vi "SLL DE Generate Plot LV2Global.vi"(7 "Option":T1=enum."Get Plot", 8 "error in (no error)":errorcluster, 9 "X-Scale":refnum<vi>, 10 "Plots":u16[](array[numeric]), 11 "Data Cluster":T3) -> (0 "error IO":errorcluster, 3 "Plot data array":T2(array[cluster]))   [LabVIEW 2009]
uses:
  Controls/SLL DE Get Plot LV2Global Parameters.ctl
  Controls/SLL DE Get Plot LV2Global Options.ctl
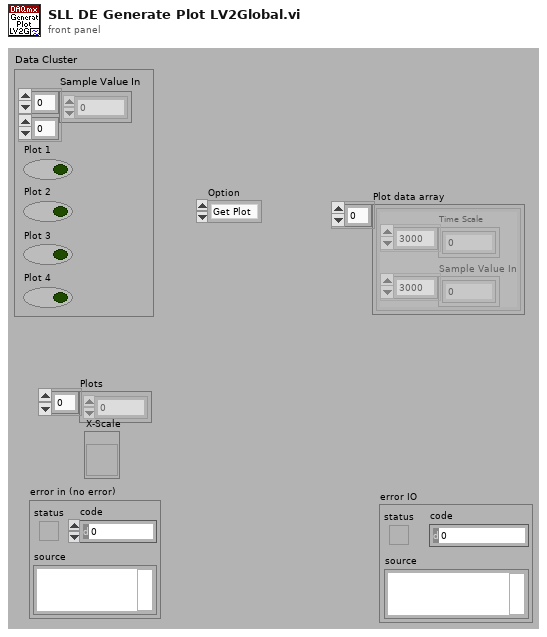
[diagram p1: front panel]
types:
  T1 = typedef "SLL DE Get Plot LV2Global Options.ctl" = enum16{"Init", "Get Plot", "Read Plot"}
  T2 = cluster{"Time Scale":sgl[], "Sample Value In":sgl[]}[]
  T3 = typedef "SLL DE Get Plot LV2Global Parameters.ctl" = cluster{"Sample Value In":sgl[][], "Plot 1":bool, "Plot 2":bool, "Plot 3":bool, "Plot 4":bool}
  T4 = cluster{"Sample Value In":sgl[], "Sample Value In":sgl[]}[]
  T5 = cluster{"Sample Value In":dbl[], "Sample Value In":sgl[]}
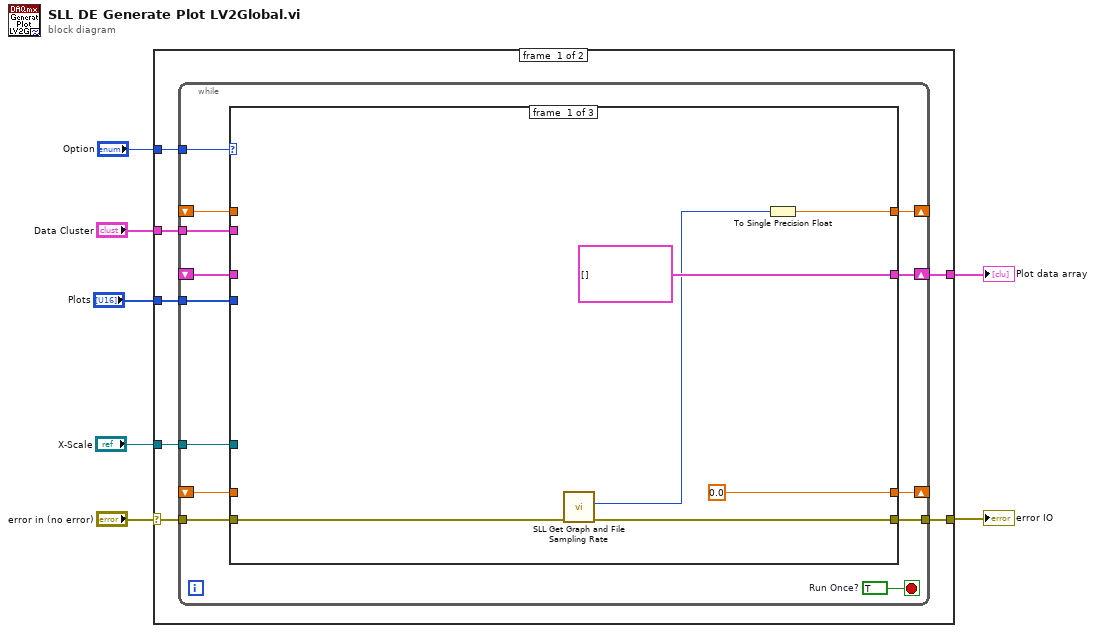
[diagram p0: block diagram]
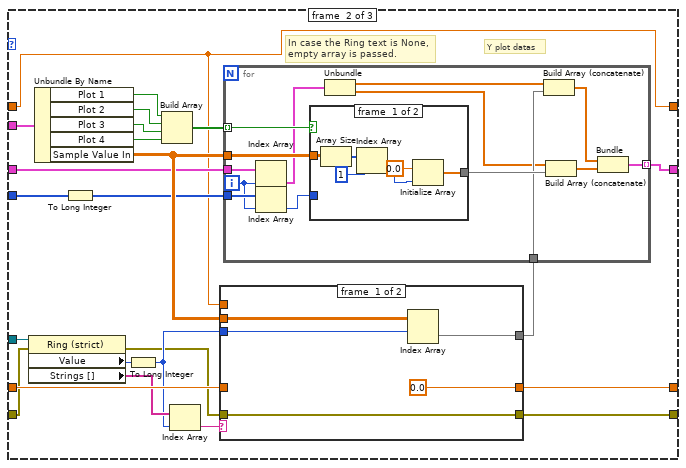
[diagram p2: hidden frame]
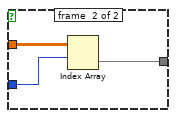
[diagram p3: hidden frame]
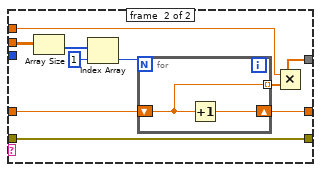
[diagram p4: hidden frame]
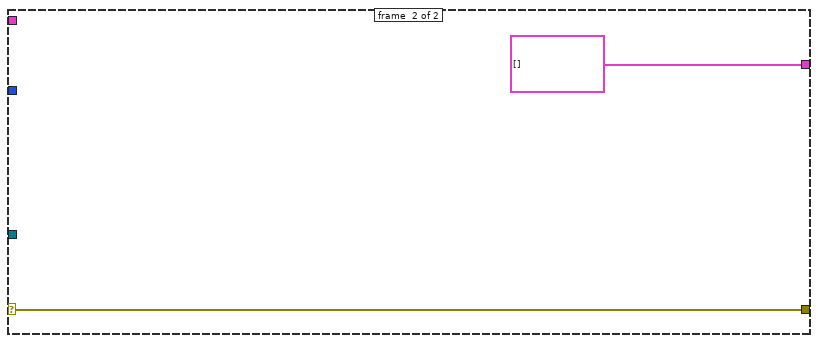
[diagram p6: hidden frame]
diagram:
  n1 = case shown="No Error" "error in (no error)" {
    selector: "error in (no error)" -> [w10 w102]
    tunnel: [w12 w102] -> w6
    tunnel: [w13 T2 []] -> w4
    tunnel: "Data Cluster" -> [w14 _]
    tunnel: "Plots" -> [w11 _]
    tunnel: "X-Scale" -> [w9 _]
    tunnel: "Option" -> [w8 _]
    frame #0 {
      n2 = while {
        tunnel: w14 -> [w27]
        tunnel: [w25] -> w12
        tunnel: w11 -> [w24]
        tunnel: w10 -> [w23]
        tunnel: w9 -> [w22]
        shift-right: [w26] -> w13
        shift-left: _ -> [w20]
        shift-right: [w19] -> _
        shift-left: _ -> [w18]
        tunnel: w8 -> [w17]
        shift-right: [w16] -> _
        shift-left: _ -> [w15]
        stop <- w21 stop-if-true
        w21 = TRUE  # Run Once?
        n3 = case shown="\"Init\", Default" w17 {
          tunnel: w27 -> [_ w56 _]
          tunnel: [T4 [] w49 w100] -> w26
          tunnel: [w30 w47 w98] -> w25
          tunnel: w24 -> [_ w46 _]
          tunnel: w23 -> [w31 w36 w98]
          tunnel: w22 -> [_ w39 _]
          tunnel: w20 -> [_ w44 w100]
          tunnel: [sgl 0.0 w42 w99] -> w19
          tunnel: w18 -> [_ w43 w99]
          tunnel: [w28 w34 w97] -> w16
          tunnel: w15 -> [_ w34 w97]
          frame #0 {
            n4 = call "SLL Get Graph and File Sampling Rate.vi"("error in (no error)"=w31) -> ("error out"=w30:errorcluster, "Graph - Interval b/w Samples"=w29:i32)  [unwired: 7 in, 2 out]
            n5 = To Single Precision Float(number=w29) -> (single precision float=w28:sgl)
          }
          frame #1 {
            # "Y plot datas"
            # "In case the Ring text is None, \nempty array is passed."
            n6 = property on="Property Node" class="Ring (strict)"(reference=w39, error in=w36) -> (error out=w35:errorcluster, "Value"=w38:u16, "Strings []"=w41:string[])  [unwired: 1 out]
            n7 = Unbundle By Name(w56) -> ("Plot 1"=w55:bool, "Plot 2"=w54:bool, "Plot 3"=w53:bool, "Plot 4"=w52:bool, "Sample Value In"=w50:sgl[][])
            n8 = To Long Integer(number=w46) -> (32bit integer=w45:i32[])
            n9 = To Long Integer(number=w38) -> (32bit integer=w37:i32)
            n10 = Build Array(w55, w54, w53, w52) -> (w51:bool[])
            n11 = Index Array(array=w41, index=w37) -> (element=w40:string)
            n12 = case shown="\"Time Scale\"" w40 {
              tunnel: [w84 w86] -> w48
              tunnel: w50 -> [w83 w93]
              tunnel: w35 -> [w82 w94]
              tunnel: [w82 w94] -> w47
              tunnel: w37 -> [w80 _]
              tunnel: w43 -> [_ w89]
              tunnel: [sgl 0.0 w87] -> w42
              tunnel: w34 -> [_ w85]
              frame #0 {
                n13 = Index Array(array=w83, index (row)=w80) -> (element=w84:sgl[])  [unwired: 1 in]
              }
              frame #1 {
                n14 = Array Size(array=w93) -> (size(s)=w92:i32[])
                n15 = Index Array(array=w92, index=1) -> (element=w91:i32)
                n16 = for {
                  N: w91 -> [_]
                  shift-right: [w96] -> w87
                  shift-left: w89 -> [w95]
                  tunnel: [w95] -> w88 mode=indexing
                  n17 = Increment(x=w95) -> (x+1=w96:sgl)
                }
                n18 = Multiply(x=w85, y=w88) -> (x*y=w86:sgl[])
              }
            }
            n19 = for {
              tunnel: w50 -> [w70]
              tunnel: w51 -> [w69] mode=indexing
              tunnel: w48 -> [w67]
              tunnel: [w66] -> w49 mode=indexing
              tunnel: w45 -> [w65]
              tunnel: w44 -> [w64]
              i -> [w57]
              n20 = Index Array(array=w64, index=w57) -> (element=w59:T5)
              n21 = Index Array(array=w65, index=w57) -> (element=w58:i32)
              n22 = case shown="False" w69 {
                tunnel: w70 -> [w75 w79]
                tunnel: w58 -> [_ w77]
                tunnel: [w74 w78] -> w68
                frame #0 {
                  n23 = Array Size(array=w75) -> (size(s)=w73:i32[])
                  n24 = Index Array(array=w73, index=1) -> (element=w72:i32)
                  n25 = Initialize Array(sgl 0.0 ("element"), w72) -> (w74:sgl[])
                }
                frame #1 {
                  n26 = Index Array(array=w79, index (row)=w77) -> (element=w78:sgl[])  [unwired: 1 in]
                }
              }
              n27 = Unbundle(w59) -> ("Sample Value In"=w62:dbl[], "Sample Value In"=w60:sgl[])
              n28 = Build Array (concatenate)(w62, w67) -> (w63:dbl[])
              n29 = Build Array (concatenate)(w60, w68) -> (w61:sgl[])
              n30 = Bundle(w63, w61) -> (w66:cluster{dbl[], sgl[]})  [unwired: 1 in]
            }
          }
          frame #2 {
          }
        }
      }
    }
    frame #1 {
    }
  }
  "error IO" <- w6
  "Plot data array" <- w4
